vi "McP grating density factor.vi"(1 "Grating Density":T1=enum."1200") -> (0 "GratingFactor":dbl format="%.2f")   [LabVIEW 2021]
uses:
  Globals and TypeDefs/Type Definitions.llb/McPherson Grating Density.ctl
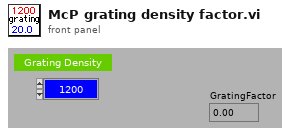
[diagram p1: front panel]
types:
  T1 = typedef "McPherson Grating Density.ctl" = enum8{"150", "300", "600", "1200", "1800"}
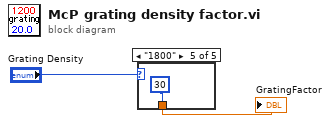
[diagram p0: block diagram]
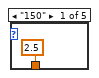
[diagram p2: hidden frame]
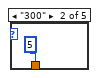
[diagram p3: hidden frame]
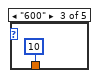
[diagram p4: hidden frame]
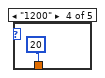
[diagram p5: hidden frame]
diagram:
  n1 = case shown="\"1800\"" "Grating Density" {
    tunnel: [2.5 5 10 20 30] -> w1
    frame "150" {
    }
    frame "300" {
    }
    frame "600" {
    }
    frame "1200" {
    }
    frame "1800" {
    }
  }
  "GratingFactor" <- w1
